vi "RSZVB Get Port Waveguide Attenuator Slope.vi"(8 "error in (no error)":errorcluster {"code" format="%.0x"}, 9 "Port (1)":i32=1, 10 "Channel (1)":i32=1, 11 "VISA session":refnum<visa-resource-name>) -> (0 "error out":errorcluster {"code" format="%.0x"}, 2 "Slope":i32, 3 "dup VISA session":refnum<visa-resource-name>)   [LabVIEW 2011]
doc: "This VI returns the slope for the linear power transfer model with 0 dB waveguide attenuation.\n\nRemote-control command(s):\nSOURce<Ch>:POWer<Pt>:CONVerter:TRANsfer:SLOPe?"
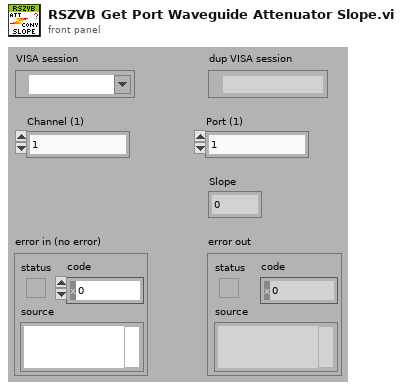
[diagram p1: front panel]
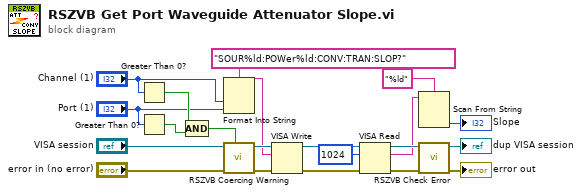
[diagram p0: block diagram]
diagram:
  n1 = Greater Than 0?(x="Channel (1)") -> (x > 0?=w15:bool)
  n2 = Greater Than 0?(x="Port (1)") -> (x > 0?=w18:bool)
  n3 = Compound Arithmetic op=AND(w15, w18) -> (w17:bool)
  n4 = Format Into String(format string="SOUR%ld:POWer%ld:CONV:TRAN:SLOP?", "Channel (1)", "Port (1)") -> (resulting string=w16:string)  [unwired: 2 in, 1 out]
  n5 = call "RSZVB Coercing Warning.vi"("In Range?"=w17, "error in (no error)"="error in (no error)", "VISA session"="VISA session") -> ("error out"=w19:errorcluster, "dup VISA session"=w20:refnum<visa-resource-name>)  [unwired: 7 in]
  n6 = VISA Write(VISA resource name=w20, write buffer=w16, error in (no error)=w19) -> (VISA resource name out=w6:refnum<visa-resource-name>, error out=w7:errorcluster)  [unwired: 1 out]
  n7 = VISA Read(VISA resource name=w6, byte count=u32 1024, error in (no error)=w7) -> (VISA resource name out=w8:refnum<visa-resource-name>, read buffer=w3:string, error out=w9:errorcluster)  [unwired: 1 out]
  n8 = Scan From String(format string="%ld", input string=w3) -> (output 1=→"Slope":i32)  [unwired: 3 in, 3 out]
  n9 = call "RSZVB Check Error.vi"("error in (no error)"=w9, "VISA session"=w8) -> ("error out"=→"error out":errorcluster, "dup VISA session"=→"dup VISA session":refnum<visa-resource-name>)  [unwired: 8 in]
